vi "Claw Roller Activate.vi"(11 "Start Rollers":bool) -> ()   [LabVIEW 2012]
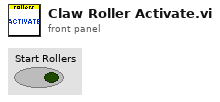
[diagram p1: front panel]
types:
  T1 = typedef "WPI_MotorControlDeviceRef.ctl" = cluster{"DeviceStatus":errorcluster, "Type":enum16{"PWM", "CAN"}, "PWM":cluster{"Digital Module":T2, "PWM Channel":T3, "DeadBand":T4}, "CAN":cluster{"Device Number":u8, "Control Mode":T5, "Semaphore":T6, "Max Vout":dbl}, "Invert":bool, "TransformRef":T7, "InvTransformRef":T7}
  T2 = typedef "FPGA_TypedefDigitalModule.ctl" = enum16{"Digital Module 1", "Digital Module 2"}
  T3 = typedef "FPGA_DIOPWMChannel.ctl" = enum8{"PWM 1", "PWM 2", "PWM 3", "PWM 4", "PWM 5", "PWM 6", "PWM 7", "PWM 8", "PWM 9", "PWM 10", "Invalid"}
  T4 = typedef "WPI_PWMDeadband.ctl" = cluster{"Name":string, "maxPositivePwm":i32, "minPositivePwm":i32, "centerPwm":i32, "maxNegativePwm":i32, "minNegativePwm":i32, "angularRange":u16}
  T5 = typedef "WPI_CANJaguar_ControlMode.ctl" = enum8{"Percent VBus", "Current", "Speed", "Position", "Voltage"}
  T6 = typedef "Semaphore RefNum" = refnum<k1>
  T7 = typedef "WPI_PWMTransform_ConPane.ctl" = refnum<vi>
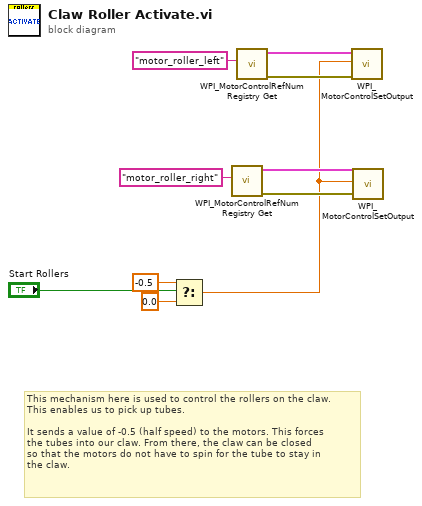
[diagram p0: block diagram]
diagram:
  # "This mechanism here is used to control the rollers on the claw. \nThis enables us to pick up tubes. \n\nIt sends a value of -0.5 (half speed) to the motors. This forces\nthe tubes into our claw. From there, the claw can be closed \nso that the motors do not have to spin for the tube to stay in \nthe claw."
  n1 = Select(t=-0.5, s="Start Rollers", f=0.0) -> (s? t:f=w2:dbl)
  n2 = call <vilib>:"WPI_MotorControlRefNum Registry Get.vi"("refnum name"="motor_roller_right") -> ("error out"=w7:errorcluster, "MotorControlDevRef"=w8:T1)  [unwired: 9 in]
  n3 = call <vilib>:"WPI_MotorControlRefNum Registry Get.vi"("refnum name"="motor_roller_left") -> ("error out"=w9:errorcluster, "MotorControlDevRef"=w10:T1)  [unwired: 9 in]
  n4 = call <vilib>:"WPI_MotorControlSetOutput.vi"("error in (no error)"=w9, "Output"=w2, "MotorControlDevRef"=w10) -> ()  [unwired: 6 in, 3 out]
  n5 = call <vilib>:"WPI_MotorControlSetOutput.vi"("error in (no error)"=w7, "Output"=w2, "MotorControlDevRef"=w8) -> ()  [unwired: 6 in, 3 out]
